vi "Read FPGA VI Reference.vi"(11 "FPGA API Concrete in":refnum<class "FPGA API Concrete.lvclass">) -> (2 "FPGA VI Reference":T1, 3 "FPGA API Concrete out":refnum<class "FPGA API Concrete.lvclass">)   [LabVIEW 2019, in "FPGA API Concrete.lvclass"]
uses:
  FPGA API Concrete.lvclass
  FPGA Ref.ctl
  FPGA API Concrete.lvclass/FPGA API Concrete.ctl
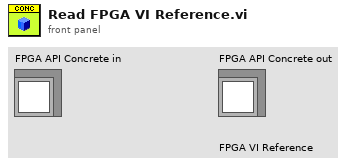
[diagram p1: front panel]
types:
  T1 = typedef "FPGA API Concrete.lvclass/FPGA Ref.ctl" = refnum<k20>
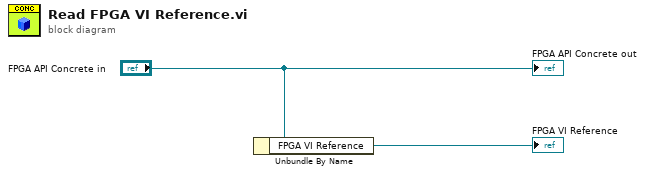
[diagram p0: block diagram]
diagram:
  n1 = Unbundle By Name("FPGA API Concrete in") -> ("FPGA VI Reference"=→"FPGA VI Reference":T1)
  "FPGA API Concrete out" <- "FPGA API Concrete in"
